vi "Failure Message.vi"() -> ()   [LabVIEW 2017, in "Transparent Assertions.Tests.lvlib" / "Assert String Not Starts With.lvlib"]
uses:
  Assert String Not Starts With.lvlib
  src/Transparent Assertions/Transparent Assertions.lvlib
panel:
  out "error out":errorcluster
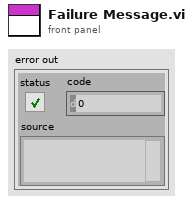
[diagram p1: front panel]
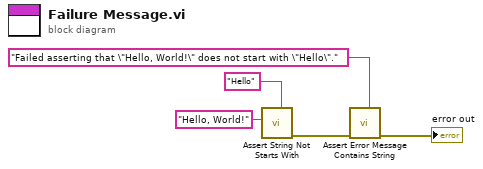
[diagram p0: block diagram]
diagram:
  n1 = call "Assert String Not Starts With.vi"("Prefix"="Hello", "String"="Hello, World!") -> ("error out"=w5:errorcluster)  [unwired: 9 in]
  n2 = call "Assert Error Message Contains String.vi"("Expected"="Failed asserting that \"Hello, World!\" does not start with \"Hello\".", "error in (no error)"=w5) -> ("error out"=→"error out":errorcluster)  [unwired: 9 in]
